vi "Conditional Frame.vi"(6 "ActiveFrame":i16, 9 "Conditions in":string[](array[string]), 10 "Disable Style":T1(ring), 11 "Diagrams":refnum<vi>[](array[refnum])) -> (2 "Class":string, 3 "Conditions out":string[](array[string]))   [LabVIEW 2023, in "VIDoc Parsing.lvlib" / "Structure Reporter.lvlib"]
uses:
  Structure Reporter.lvlib
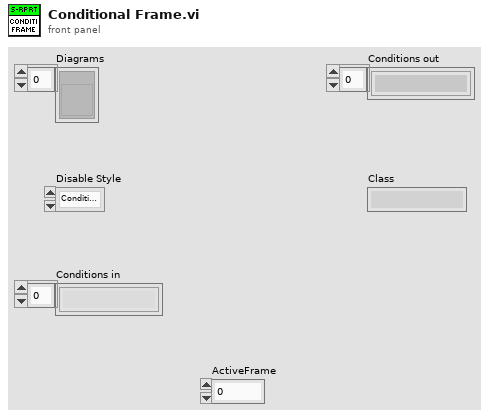
[diagram p1: front panel]
types:
  T1 = enum32{"Conditional Disable Style", "Diagram Disable Style", "Type Specialization Style"}
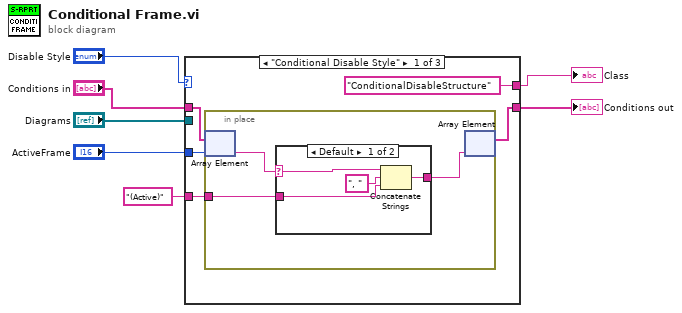
[diagram p0: block diagram]
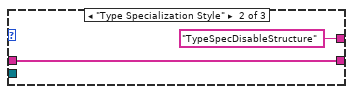
[diagram p3: hidden frame]
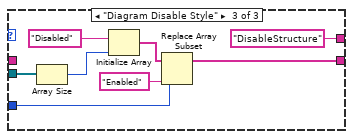
[diagram p4: hidden frame]
diagram:
  n1 = case shown="\"Conditional Disable Style\"" "Disable Style" {
    tunnel: "Conditions in" -> [w11 w22 _]
    tunnel: "ActiveFrame" -> [w10 _ w26]
    tunnel: [w9 w22 w27] -> w4
    tunnel: "Diagrams" -> [_ _ w24]
    tunnel: ["ConditionalDisableStructure" "TypeSpecDisableStructure" "DisableStructure"] -> w6
    tunnel: "(Active)" -> [w8 _ _]
    frame "Conditional Disable Style" {
      n2 = in-place {
        in-place-border: w8 -> [w13]
        n3 = in-place-array #1(w11, w10) -> (w15:string)
        n4 = case shown="Default" w15 {
          selector: w15 -> [w19 _]
          tunnel: [w17 w20] -> w14
          tunnel: w13 -> [w18 w20]
          frame Default {
            n5 = Concatenate Strings(w19, ", " ("string"), w18) -> (w17:string)
          }
          frame "" {
          }
        }
        n6 = in-place-array #1(w14) -> (w9:string[])  [unwired: 1 out]
      }
    }
    frame "Type Specialization Style" {
    }
    frame "Diagram Disable Style" {
      n7 = Array Size(array=w24) -> (size(s)=w30:i32)
      n8 = Initialize Array("Disabled", w30) -> (w28:string[])
      n9 = Replace Array Subset(array=w28, new element="Enabled", index=w26) -> (w27:string[])
    }
  }
  "Class" <- w6
  "Conditions out" <- w4
